vi "Execute.vi"(8 "error in":errorcluster, 10 "Change Laser Frequency in":refnum<class "Change PAS Laser Parameters.lvclass">, 11 "Object In":refnum<class>) -> (0 "error out":errorcluster, 3 "Object Out":refnum<class>)   [LabVIEW 2014, in "Change PAS Laser Parameters.lvclass"]
doc: "Abstract method for accomplishing the execution of a command directed to an instrument object on the wire."
uses:
  Change PAS Laser Parameters.lvclass
  Instrument/ePAS.lvclass
  FPGA/Session/Exscalabar FPGA.lvclass
  <vilib>/rvi/interface/nirviReadWriteControl/nirviReadWriteControl.xnode
  FPGA/R FPGA Ref.ctl
  ePAS Library.lvlib
  NiFpgaLv.dll
  <vilib>/Utility/error.llb/Error Cluster From Error Code.vi
  <vilib>/rvi/errors/niLvFpgaAdjustHostInterfaceError.vi
  reusable/Instrument/Instrument.lvclass
  reusable/Session APIs/Session Log/System Log.lvclass
  FPGA Bitfiles/FPGAServerV2.lvbitx
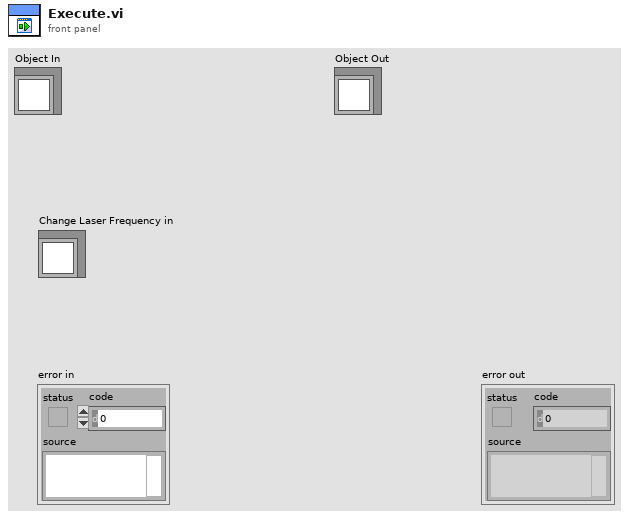
[diagram p1: front panel]
types:
  T1 = typedef "Session - Root.lvclass/Session Handle.ctl" = refnum<data-value>
  T2 = typedef "ePAS Library.lvlib/R FPGA Ref.ctl" = refnum<k20>
  T3 = cluster{"f0":fxp<+,32,0>, "Scale":fxp<+,14,1>, i16, "Modulation":enum8{"Sine", "Square"}}
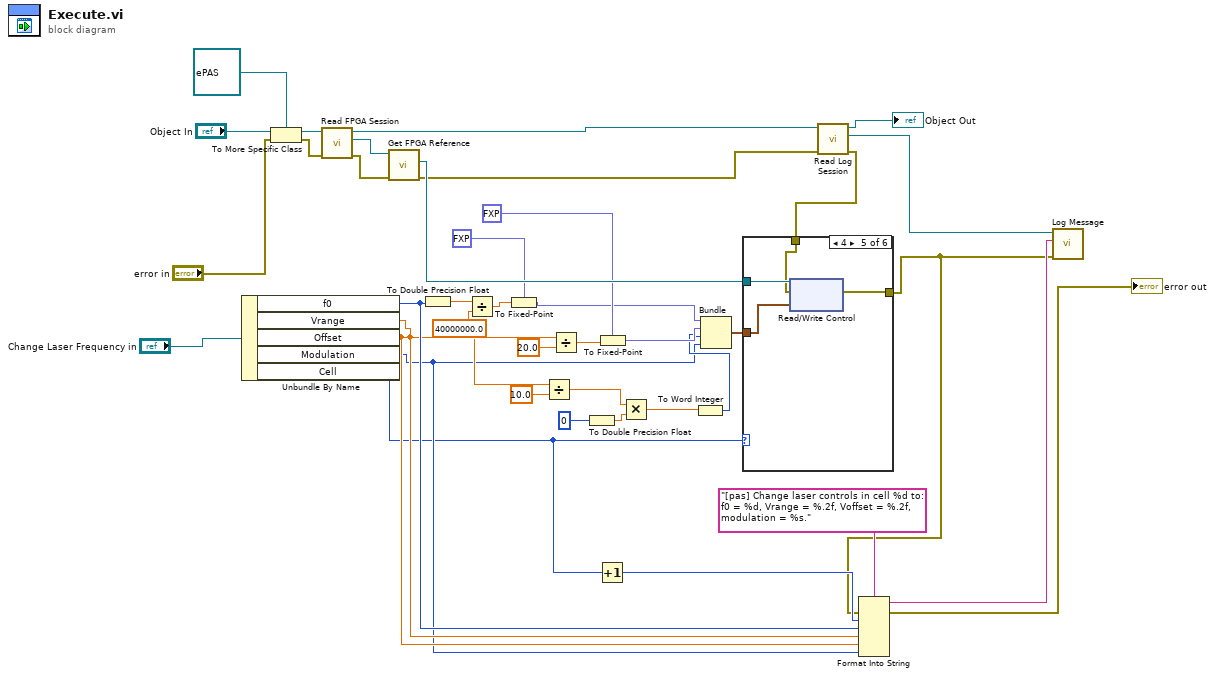
[diagram p0: block diagram]
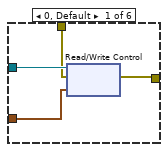
[diagram p2: hidden frame]
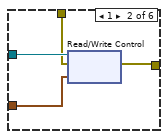
[diagram p3: hidden frame]
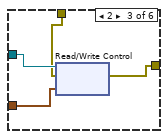
[diagram p4: hidden frame]
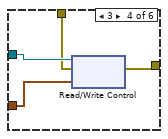
[diagram p5: hidden frame]
diagram:
  n1 = Unbundle By Name("Change Laser Frequency in") -> ("f0"=w9:u16, "Vrange"=w8:sgl, "Offset"=w7:sgl, "Modulation"=w6:enum8{"Sine", "Square"}, "Cell"=w4:u8)
  n2 = To More Specific Class(target class=refnum<class "ePAS.lvclass"> refnum ("ePAS"), reference="Object In", error in="error in") -> (specific class reference=w38:refnum<class "ePAS.lvclass">, error out=w37:errorcluster)
  n3 = call "Read FPGA Session.vi"("error in (no error)"=w37, "ePAS in"=w38) -> ("error out"=w34:errorcluster, "Session Handle"=w36:T1, "ePAS out"=w15:refnum<class "ePAS.lvclass">)  [unwired: 7 in]
  n4 = call "Get FPGA Reference.vi"("error in"=w34, "Session In"=w36) -> ("error out"=w12:errorcluster, "Ex FPGA Ref"=w32:T2)  [unwired: 7 in, 1 out]
  n5 = To Double Precision Float(number=w9) -> (double precision float=w31:dbl)
  n6 = Divide(x=w31, y=40000000.0) -> (x/y=w29:dbl)
  n7 = To Fixed-Point(fixed-point type=fxp<+,32,0> 0.0 ("f0"), number=w29) -> (fixed-point=w19:fxp<+,32,0>)
  n8 = Divide(x=w7, y=sgl 10.0) -> (x/y=w21:sgl)
  n9 = Divide(x=w8, y=sgl 20.0) -> (x/y=w26:sgl)
  n10 = To Double Precision Float(number=i16 0) -> (double precision float=w22:dbl)
  n11 = Increment(x=w4) -> (x+1=w3:u8)
  n12 = To Fixed-Point(fixed-point type=fxp<+,14,1> 0.0 ("Scale"), number=w26) -> (fixed-point=w18:fxp<+,14,1>)
  n13 = Multiply(x=w21, y=w22) -> (x*y=w20:dbl)
  n14 = To Word Integer(number=w20) -> (16bit integer=w17:i16)
  n15 = Bundle("f0"=w19, "Scale"=w18, w17, "Modulation"=w6) -> (w16:T3)  [unwired: 1 in]
  n16 = call "Read Log Session.vi"("error in (no error)"=w12, "Instrument in"=w15) -> ("error out"=w11:errorcluster, "Session Handle"=w13:T1, "Instrument out"=→"Object Out":refnum<class "Instrument.lvclass">)  [unwired: 7 in]
  n17 = case shown="4" w4 {
    tunnel: w32 -> [w44 w48 w52 w56 w60 _]
    tunnel: w16 -> [w43 w47 w49 w55 w57 _]
    tunnel: w11 -> [w41 w46 w51 w54 w59 w61]
    tunnel: [w42 w45 w50 w53 w58 w61] -> w2
    frame 0, Default {
      n18 = xnode "Read/Write Control"("FPGA VI Reference In"=w44, "error in"=w41, "Cell 1"=w43) -> ("error out"=w42:errorcluster)  [unwired: 1 out]
    }
    frame 1 {
      n19 = xnode "Read/Write Control"("FPGA VI Reference In"=w48, "error in"=w46, "Cell 2"=w47) -> ("error out"=w45:errorcluster)  [unwired: 1 out]
    }
    frame 2 {
      n20 = xnode "Read/Write Control"("FPGA VI Reference In"=w52, "error in"=w51, "Cell 3"=w49) -> ("error out"=w50:errorcluster)  [unwired: 1 out]
    }
    frame 3 {
      n21 = xnode "Read/Write Control"("FPGA VI Reference In"=w56, "error in"=w54, "Cell 4"=w55) -> ("error out"=w53:errorcluster)  [unwired: 1 out]
    }
    frame 4 {
      n22 = xnode "Read/Write Control"("FPGA VI Reference In"=w60, "error in"=w59, "Cell 5"=w57) -> ("error out"=w58:errorcluster)  [unwired: 1 out]
    }
    frame 5 {
    }
  }
  n23 = Format Into String(format string="[pas] Change laser controls in cell %d to: f0 = %d, Vrange = %.2f, Voffset = %.2f, modulation = %s.", error in=w2, w3, w9, w8, w7, w6) -> (resulting string=w5:string, error out=→"error out":errorcluster)  [unwired: 1 in]
  n24 = call "Log Message.vi"("error in"=w2, "MSG In"=w5, "session in"=w13) -> ()  [unwired: 7 in, 2 out]
